vi "encrypt.vi"(0 "HGF_GPG":refnum<class "HGF_GPG.lvclass">, 1 "options file":path, 2 "keyringfile":path, 3 "Sec keyringfile":path, 4 "string in":string, 5 "error in (no error)":errorcluster, 7 "reveicer array":string[](array[string]), 8 "Trust DB":path, 9 "receiver":string) -> (10 "dup Trust DB":path, 11 "success":bool=TRUE, 13 "data error":bool, 14 "dup HGF_GPG":refnum<class "HGF_GPG.lvclass">, 15 "dup options file":path, 16 "dup keyringfile":path, 17 "dup Sec keyringfile":path, 18 "String out":string, 19 "error out":errorcluster)   [LabVIEW 2012, in "HGF_GPG.lvlib" / "HGF_GPG.lvclass"]
doc: "Encrypt a string. Only receiver in the list can decrypt the string."
uses:
  HGF_GPG.lvclass
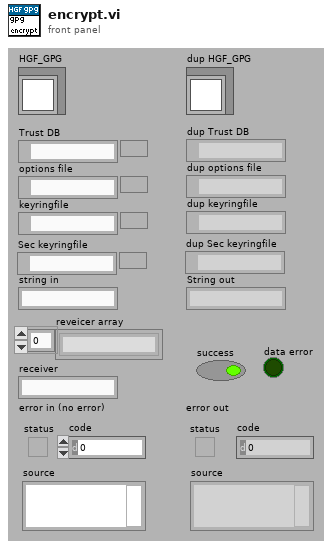
[diagram p1: front panel]
types:
  T1 = enum16{"open", "replace", "create", "open or create", "replace or create", "replace or create with confirmation"}
  T2 = enum16{"encrypt", "decrypt", "sign", "verify", "sign & encrypt", "verify & decrypt"}
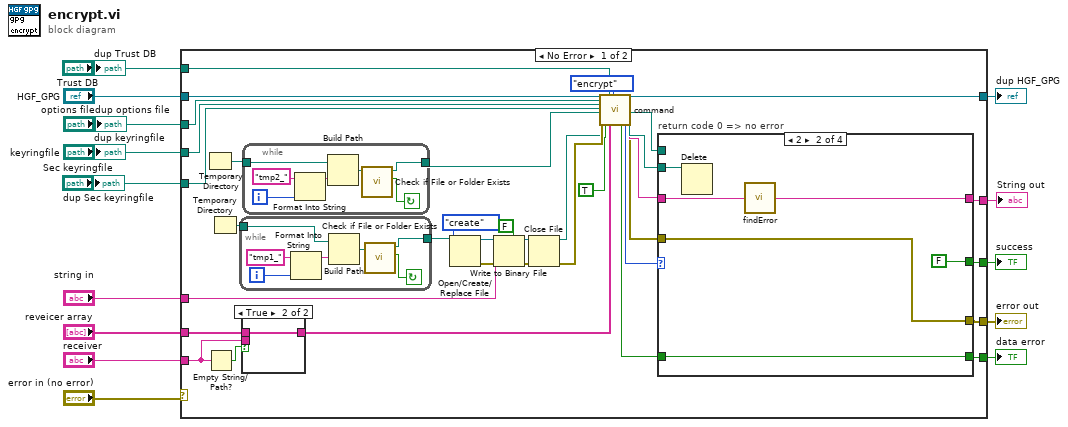
[diagram p0: block diagram]
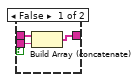
[diagram p2: hidden frame]
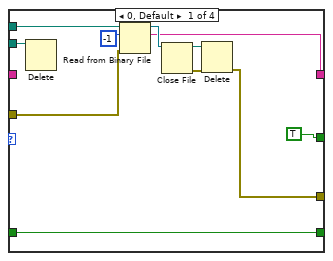
[diagram p3: hidden frame]
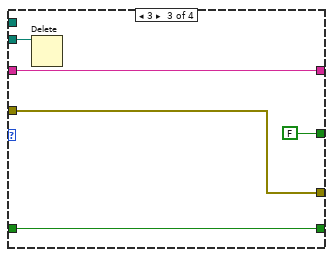
[diagram p4: hidden frame]
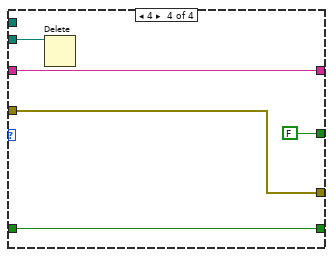
[diagram p5: hidden frame]
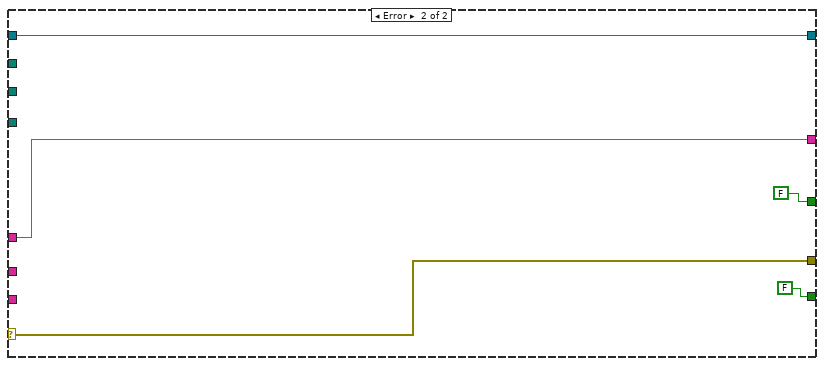
[diagram p6: hidden frame]
diagram:
  n1 = case shown="No Error" "error in (no error)" {
    selector: "error in (no error)" -> [_ w98]
    tunnel: [w47 w99] -> w12
    tunnel: "HGF_GPG" -> [w48 w99]
    tunnel: "receiver" -> [w27 _]
    tunnel: [w39 w98] -> w8
    tunnel: "string in" -> [w46 w97]
    tunnel: [w38 w97] -> w9
    tunnel: [w31 FALSE ("data error?")] -> w7
    tunnel: [w30 FALSE] -> w6
    tunnel: "reveicer array" -> [w29 _]
    tunnel: "options file" -> [w20 _]
    tunnel: "keyringfile" -> [w19 _]
    tunnel: "Sec keyringfile" -> [w16 _]
    tunnel: "Trust DB" -> [w15 _]
    frame No Error {
      n2 = Temporary Directory() -> (w33:path)
      n3 = Empty String/Path?(string/path=w27) -> (empty?=w28:bool)
      n4 = Temporary Directory() -> (w34:path)
      n5 = while {
        tunnel: [w94] -> w37
        tunnel: w34 -> [w92]
        i -> [w90]
        stop <- w93 continue-if-true
        n6 = Format Into String(initial string="tmp1_" ("name or relative path"), w90) -> (resulting string=w89:string)  [unwired: 2 in, 1 out]
        n7 = Build Path(base path=w92, name or relative path=w89) -> (appended path=w88:path)
        n8 = call <vilib>:"Check if File or Folder Exists.vi"("path"=w88) -> ("file or folder exists?"=w93:bool, "dup path"=w94:path)  [unwired: 1 in, 8 out]
      }
      n9 = case shown="True" w28 {
        tunnel: [w52 w53] -> w23
        tunnel: w29 -> [w51 w53]
        tunnel: w27 -> [w50 _]
        frame False {
          n10 = Build Array (concatenate)(w51, w50) -> (w52:string[])
        }
        frame True {
        }
      }
      n11 = while {
        tunnel: w33 -> [w87]
        tunnel: [w85] -> w21
        i -> [w83]
        stop <- w84 continue-if-true
        n12 = Format Into String(initial string="tmp2_" ("name or relative path"), w83) -> (resulting string=w82:string)  [unwired: 2 in, 1 out]
        n13 = Build Path(base path=w87, name or relative path=w82) -> (appended path=w86:path)
        n14 = call <vilib>:"Check if File or Folder Exists.vi"("path"=w86) -> ("file or folder exists?"=w84:bool, "dup path"=w85:path)  [unwired: 1 in, 8 out]
      }
      n15 = Open/Create/Replace File(file path (use dialog)=w37, operation (0:open)=T1."create") -> (refnum out=w36:refnum<file>, error out=w32:errorcluster)  [unwired: 1 in, 4 out]
      n16 = Write to Binary File(file (use dialog)=w36, data=w46, error in=w32, 5:FALSE ("prepend array or string size? (T)")) -> (refnum out=w45:refnum<file>, error out=w44:errorcluster)  [unwired: 3 out]
      n17 = Close File(refnum=w45, error in=w44) -> (path=w22:path, error out=w43:errorcluster)
      n18 = call-dynamic "command.vi"("HGF_GPG"=w48, "options file"=w20, "keyringfile"=w19, "Sec keyringfile"=w16, "targetfile"=w21, "sourcefile"=w22, "error in (no error)"=w43, "overwrite? (t)"=TRUE ("overwrite?"), "Trust DB"=w15, "reveiver"=w23, "task"=T2."encrypt") -> ("data error"=w40:bool, "return code"=w18:i32, "dup HGF_GPG"=w47:refnum<class "HGF_GPG.lvclass">, "dup targetfile"=w17:path, "dup sourcefile"=w49:path, "standard error"=w42:string, "error out"=w41:errorcluster)  [unwired: 2 in, 8 out]
      n19 = case "return code 0 => no error" shown="2" w18 {
        tunnel: w42 -> [_ w68 w75 w79]
        tunnel: w49 -> [w64 w69 w73 w78]
        tunnel: w41 -> [w63 w70 w74 w80]
        tunnel: w40 -> [w56 w65 w71 w76]
        tunnel: [w60 w70 w74 w80] -> w39
        tunnel: [w58 w67 w75 w79] -> w38
        tunnel: [w56 w65 w71 w76] -> w31
        tunnel: [TRUE FALSE FALSE FALSE] -> w30
        tunnel: w17 -> [w54 _ _ _]
        frame 0, Default {
          n20 = Delete(path (use dialog)=w64) -> ()  [unwired: 1 in, 6 out]
          n21 = Read from Binary File(8:w63, 10:-1 ("count (1)"), 11:w54) -> (2:w58:string, 3:w62:refnum<file>)  [unwired: 5 out]
          n22 = Close File(refnum=w62) -> (path=w59:path, error out=w61:errorcluster)  [unwired: 1 in]
          n23 = Delete(path (use dialog)=w59, error in=w61) -> (error out=w60:errorcluster)  [unwired: 5 out]
        }
        frame 2 {
          n24 = Delete(path (use dialog)=w69) -> ()  [unwired: 1 in, 6 out]
          n25 = call "findError.vi"("error string in"=w68) -> ("error out"=w67:string)
        }
        frame 3 {
          n26 = Delete(path (use dialog)=w73) -> ()  [unwired: 1 in, 6 out]
        }
        frame 4 {
          n27 = Delete(path (use dialog)=w78) -> ()  [unwired: 1 in, 6 out]
        }
      }
    }
    frame Error {
    }
  }
  "error out" <- w8
  "dup HGF_GPG" <- w12
  "String out" <- w9
  "success" <- w6
  "data error" <- w7
  "dup options file" <- "options file"
  "dup keyringfile" <- "keyringfile"
  "dup Sec keyringfile" <- "Sec keyringfile"
  "dup Trust DB" <- "Trust DB"
